vi "BallLoaderNew.vi"   [LabVIEW 2011]
uses:
  Robot Global Data.vi
types:
  T1 = typedef "WPI_MotorControlDeviceRef.ctl" = cluster{"DeviceStatus":errorcluster, "Type":enum16{"PWM", "CAN"}, "PWM":cluster{"Digital Module":T2, "PWM Channel":T3, "DeadBand":T4}, "CAN":cluster{"Device Number":u8, "Control Mode":T5, "Semaphore":T6, "Max Vout":dbl}, "Invert":bool, "TransformRef":T7, "InvTransformRef":T7}
  T2 = typedef "FPGA_TypedefDigitalModule.ctl" = enum16{"Digital Module 1", "Digital Module 2"}
  T3 = typedef "FPGA_DIOPWMChannel.ctl" = enum8{"PWM 1", "PWM 2", "PWM 3", "PWM 4", "PWM 5", "PWM 6", "PWM 7", "PWM 8", "PWM 9", "PWM 10", "Invalid"}
  T4 = typedef "WPI_PWMDeadband.ctl" = cluster{"Name":string, "maxPositivePwm":i32, "minPositivePwm":i32, "centerPwm":i32, "maxNegativePwm":i32, "minNegativePwm":i32, "angularRange":u16}
  T5 = typedef "WPI_CANJaguar_ControlMode.ctl" = enum8{"Percent VBus", "Current", "Speed", "Position", "Voltage"}
  T6 = typedef "Semaphore RefNum" = refnum<k1>
  T7 = typedef "WPI_PWMTransform_ConPane.ctl" = refnum<vi>
  T8 = typedef "WPI_DigitalInputDevRef.ctl" = cluster{"DevStatus":errorcluster, "DIO Channel":T9, "Digital Module":T2}
  T9 = typedef "FPGA_DIOChannel.ctl" = enum8{"DIO 1", "DIO 2", "DIO 3", "DIO 4", "DIO 5", "DIO 6", "DIO 7", "DIO 8", "DIO 9", "DIO 10", "DIO 11", "DIO 12", "DIO 13", "DIO 14", "Invalid"}
  T10 = enum16{"Shoot", "Load", "Arm", "Nothing", "Reverse", "ShootAll"}
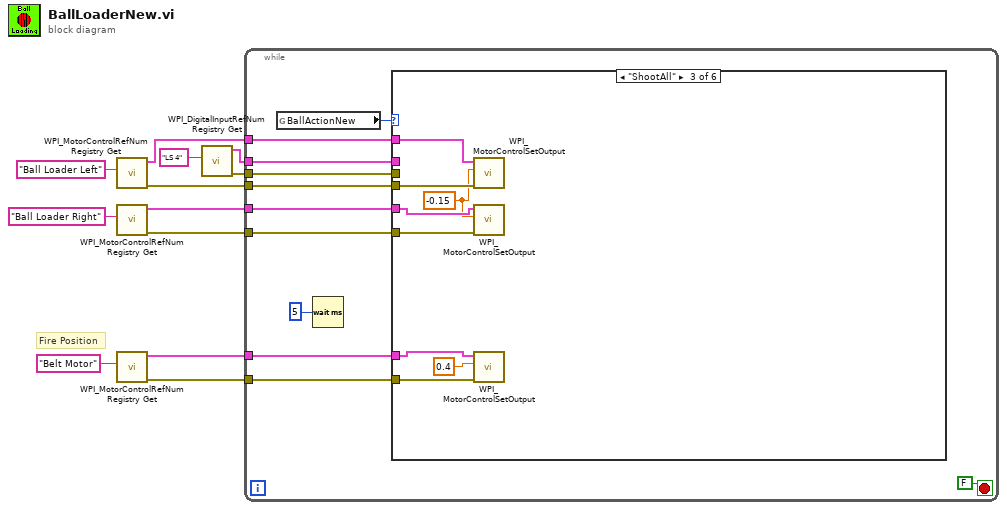
[diagram p0: block diagram]
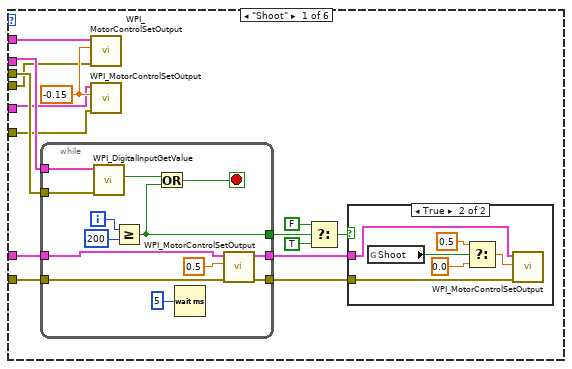
[diagram p2: hidden frame]
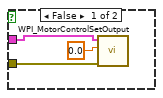
[diagram p3: hidden frame]
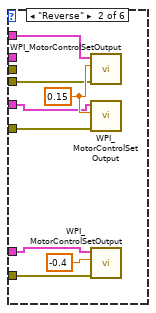
[diagram p4: hidden frame]
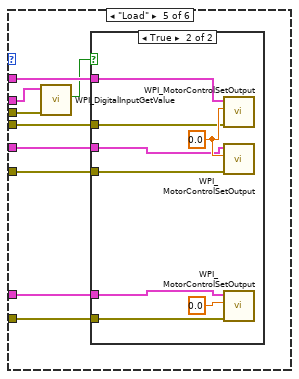
[diagram p6: hidden frame]
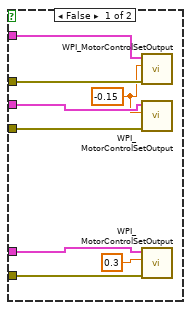
[diagram p7: hidden frame]
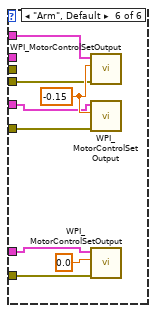
[diagram p8: hidden frame]
diagram:
  # "Fire Position"
  n1 = call <vilib>:"WPI_MotorControlRefNum Registry Get.vi"("refnum name"="Ball Loader Left") -> ("error out"=w7:errorcluster, "MotorControlDevRef"=w8:T1)  [unwired: 9 in]
  n2 = call <vilib>:"WPI_MotorControlRefNum Registry Get.vi"("refnum name"="Ball Loader Right") -> ("error out"=w9:errorcluster, "MotorControlDevRef"=w10:T1)  [unwired: 9 in]
  n3 = call <vilib>:"WPI_MotorControlRefNum Registry Get.vi"("refnum name"="Belt Motor") -> ("error out"=w5:errorcluster, "MotorControlDevRef"=w4:T1)  [unwired: 9 in]
  n4 = call <vilib>:"WPI_DigitalInputRefNum Registry Get.vi"("refnum name"="LS 4") -> ("error out"=w2:errorcluster, "DigitalInputDevRef"=w3:T8)  [unwired: 9 in]
  n5 = while {
    tunnel: w10 -> [w23]
    tunnel: w9 -> [w22]
    tunnel: w8 -> [w21]
    tunnel: w7 -> [w20]
    tunnel: w5 -> [w19]
    tunnel: w4 -> [w18]
    tunnel: w3 -> [w17]
    tunnel: w2 -> [w16]
    stop <- FALSE stop-if-true
    n6 = global read "Robot Global Data.vi" "BallActionNew"() -> (w15:T10)
    n7 = Wait (ms)(milliseconds to wait=u32 5) -> ()  [unwired: 1 out]
    n8 = case shown="\"ShootAll\"" w15 {
      tunnel: w18 -> [w36 w66 w72 _ w78 w107]
      tunnel: w19 -> [w35 w65 w71 _ w77 w106]
      tunnel: w23 -> [w25 w64 w75 _ w85 w105]
      tunnel: w22 -> [w24 w63 w73 _ w84 w104]
      tunnel: w21 -> [w27 w62 w76 _ w83 w103]
      tunnel: w20 -> [w26 w61 w74 _ w82 w102]
      tunnel: w16 -> [w37 _ _ _ w81 _]
      tunnel: w17 -> [w38 _ _ _ w80 _]
      frame "Shoot" {
        w28 = -0.15 ("Output")
        n9 = while {
          tunnel: w38 -> [w60]
          tunnel: w37 -> [w59]
          tunnel: w36 -> [w54]
          tunnel: w35 -> [w53]
          tunnel: [w52] -> w34
          tunnel: [w51] -> w33
          tunnel: [w50] -> w32
          i -> [w49]
          stop <- w56 stop-if-true
          n10 = call <vilib>:"WPI_DigitalInputGetValue.vi"("error in (no error)"=w59, "DigitalInputDevRef"=w60) -> ("Value"=w57:bool)  [unwired: 7 in, 2 out]
          n11 = Greater Or Equal?(x=w49, y=200) -> (x >= y?=w50:bool)
          n12 = Or(x=w57, y=w50) -> (x .or. y?=w56:bool)
          n13 = Wait (ms)(milliseconds to wait=u32 5) -> ()  [unwired: 1 out]
          n14 = call <vilib>:"WPI_MotorControlSetOutput.vi"("error in (no error)"=w53, "Output"=0.5, "MotorControlDevRef"=w54) -> ("error out"=w51:errorcluster, "MotorControlDevRef"=w52:T1)  [unwired: 7 in]
        }
        n15 = call <vilib>:"WPI_MotorControlSetOutput.vi"("error in (no error)"=w26, "Output"=w28, "MotorControlDevRef"=w27) -> ()  [unwired: 7 in, 2 out]
        n16 = call <vilib>:"WPI_MotorControlSetOutput.vi"("error in (no error)"=w24, "Output"=w28, "MotorControlDevRef"=w25) -> ()  [unwired: 7 in, 2 out]
        n17 = Select(t=FALSE, s=w32, f=TRUE) -> (s? t:f=w29:bool)
        n18 = case shown="True" w29 {
          tunnel: w34 -> [w41 w46]
          tunnel: w33 -> [w40 w45]
          frame False {
            n19 = call <vilib>:"WPI_MotorControlSetOutput.vi"("error in (no error)"=w40, "Output"=0.0, "MotorControlDevRef"=w41) -> ()  [unwired: 7 in, 2 out]
          }
          frame True {
            n20 = global read "Robot Global Data.vi" "Shoot"() -> (w47:bool)
            n21 = Select(t=0.5, s=w47, f=0.0) -> (s? t:f=w42:dbl)
            n22 = call <vilib>:"WPI_MotorControlSetOutput.vi"("error in (no error)"=w45, "Output"=w42, "MotorControlDevRef"=w46) -> ()  [unwired: 7 in, 2 out]
          }
        }
      }
      frame "Reverse" {
        w68 = 0.15 ("Output")
        n23 = call <vilib>:"WPI_MotorControlSetOutput.vi"("error in (no error)"=w61, "Output"=w68, "MotorControlDevRef"=w62) -> ()  [unwired: 7 in, 2 out]
        n24 = call <vilib>:"WPI_MotorControlSetOutput.vi"("error in (no error)"=w63, "Output"=w68, "MotorControlDevRef"=w64) -> ()  [unwired: 7 in, 2 out]
        n25 = call <vilib>:"WPI_MotorControlSetOutput.vi"("error in (no error)"=w65, "Output"=-0.4, "MotorControlDevRef"=w66) -> ()  [unwired: 7 in, 2 out]
      }
      frame "ShootAll" {
        w70 = -0.15 ("Output")
        n26 = call <vilib>:"WPI_MotorControlSetOutput.vi"("error in (no error)"=w74, "Output"=w70, "MotorControlDevRef"=w76) -> ()  [unwired: 7 in, 2 out]
        n27 = call <vilib>:"WPI_MotorControlSetOutput.vi"("error in (no error)"=w73, "Output"=w70, "MotorControlDevRef"=w75) -> ()  [unwired: 7 in, 2 out]
        n28 = call <vilib>:"WPI_MotorControlSetOutput.vi"("error in (no error)"=w71, "Output"=0.4, "MotorControlDevRef"=w72) -> ()  [unwired: 7 in, 2 out]
      }
      frame "Nothing" {
      }
      frame "Load" {
        n29 = call <vilib>:"WPI_DigitalInputGetValue.vi"("error in (no error)"=w81, "DigitalInputDevRef"=w80) -> ("Value"=w79:bool)  [unwired: 7 in, 2 out]
        n30 = case shown="True" w79 {
          tunnel: w85 -> [w93 w96]
          tunnel: w84 -> [w92 w97]
          tunnel: w83 -> [w91 w94]
          tunnel: w82 -> [w90 w95]
          tunnel: w78 -> [w87 w99]
          tunnel: w77 -> [w86 w98]
          frame False {
            w89 = -0.15 ("Output")
            n31 = call <vilib>:"WPI_MotorControlSetOutput.vi"("error in (no error)"=w90, "Output"=w89, "MotorControlDevRef"=w91) -> ()  [unwired: 7 in, 2 out]
            n32 = call <vilib>:"WPI_MotorControlSetOutput.vi"("error in (no error)"=w92, "Output"=w89, "MotorControlDevRef"=w93) -> ()  [unwired: 7 in, 2 out]
            n33 = call <vilib>:"WPI_MotorControlSetOutput.vi"("error in (no error)"=w86, "Output"=0.3, "MotorControlDevRef"=w87) -> ()  [unwired: 7 in, 2 out]
          }
          frame True {
            w101 = 0.0 ("Output")
            n34 = call <vilib>:"WPI_MotorControlSetOutput.vi"("error in (no error)"=w95, "Output"=w101, "MotorControlDevRef"=w94) -> ()  [unwired: 7 in, 2 out]
            n35 = call <vilib>:"WPI_MotorControlSetOutput.vi"("error in (no error)"=w97, "Output"=w101, "MotorControlDevRef"=w96) -> ()  [unwired: 7 in, 2 out]
            n36 = call <vilib>:"WPI_MotorControlSetOutput.vi"("error in (no error)"=w98, "Output"=0.0, "MotorControlDevRef"=w99) -> ()  [unwired: 7 in, 2 out]
          }
        }
      }
      frame "Arm", Default {
        w108 = -0.15 ("Output")
        n37 = call <vilib>:"WPI_MotorControlSetOutput.vi"("error in (no error)"=w102, "Output"=w108, "MotorControlDevRef"=w103) -> ()  [unwired: 7 in, 2 out]
        n38 = call <vilib>:"WPI_MotorControlSetOutput.vi"("error in (no error)"=w104, "Output"=w108, "MotorControlDevRef"=w105) -> ()  [unwired: 7 in, 2 out]
        n39 = call <vilib>:"WPI_MotorControlSetOutput.vi"("error in (no error)"=w106, "Output"=0.0, "MotorControlDevRef"=w107) -> ()  [unwired: 7 in, 2 out]
      }
    }
  }
